vi "AODScanner.vi"() -> ()   [LabVIEW 2011]
uses:
  <vilib>/userdefined/High Color/nirio_resource_hc.ctl
  AODAcq/AODAcq.lvclass
  <vilib>/DAQmx/write.llb/DAQmx Write (Analog DBL 1Chan 1Samp).vi
  <vilib>/DAQmx/read.llb/DAQmx Read (Analog Wfm 1Chan NSamp).vi
  <vilib>/DAQmx/miscellaneous.llb/DAQmx Fill In Error Info.vi
  <vilib>/Utility/error.llb/Error Cluster From Error Code.vi
  <vilib>/rvi/errors/niLvFpgaAdjustHostInterfaceError.vi
  <vilib>/rvi/interface/nirviReadWriteControl/nirviReadWriteControl.xnode
  FPGA_Control/AODRef.ctl
  FPGA_Control/FPGA Bitfiles/AODControl_FPGATarget_5751Acquire_038F9455.lvbitx
  FPGA_Control/AOD Control (FPGA).vi
  NiFpgaLv.dll
panel:
  out "# elements in queue":i32
  out "Waveform Chart":waveform(dbl)(graph)
  out "Ephys":bool
  in  "TraceElements":u32=10000
  out "ScanProgress":dbl(slide) scale=0.0..1.0
  in  "Abort":bool
  out "Progress":dbl(slide) scale=0.0..1.0
  in  "SweepSettings":bool
  in  "stop":bool
  in  "Power":dbl(slide) min=0.0 max=5.0 step=0.1 scale=0.0..2.5
  out "Point Scanning":bool
  out "Volume Scanning":bool
  in  "Tab Control":enum32{"Setup", "Volume", "Traces", "Motion"}(tab)=enum."Volume"
  in  "Ephys":bool
  in  "Motion rate (Hz)":dbl
  in  "ClearPoints":bool
  in  "Recording Settings":T1
  in  "Scan Settings (um)":T2={"XStart"=-100, "XEnd"=100, "XNum"=250, "YStart"=-100, "YEnd"=100, "YNum"=250, "ZStart"=-50, "ZEnd"=50, "ZNum"=30}
  in  "RIO Device":T3="RIO0"
  in  "Objective":enum16{"20x Olympus"}(ring)
  in  "Scan Time (s)":dbl=300.0
  in  "Volume Reps":i32=1 min=1 max=10000
  in  "Volume":bool
  in  "Scan":bool
  in  "Decimate":bool
  out "Motion points":u32
  in  "MaxThreshold":dbl=1.0
  out "Number selected":u32
  in  "Number of cells":u32=200
  in  "Threshold":dbl=0.1
  in  "Max":dbl(slide)=700000.0 scale=0.0..1310720.0
  out "ImCh2":T4(plugin-control)
  out "ImCh1":T4(plugin-control)
  in  "Section":dbl min=0.0 max=29.0 step=1.0
  in  "Segment":bool
  out "Motion Increment":u32
  in  "DisplayVol":bool=TRUE
  out "Motion Ch1":T4(plugin-control)
  out "Ephys":waveform(dbl)[](graph)
  out "Traces":waveform(dbl)[](graph)
  in  "Down Rate":i32=500
  in  "Spacing":dbl=100.0
  out "Motion Ch2":T4(plugin-control)
  out "Finished":bool
  out "Stopped":bool
  out "AODAcq out":refnum<class "AODAcq.lvclass">
  in  "Debug":bool
  in  "GridPoints":u16=10
  out "Scan Settings":T2
  out "VolData":u8[][](array[numeric])
  in  "VolumeElements":u32=10000
  in  "Points":i32[][](array[numeric])
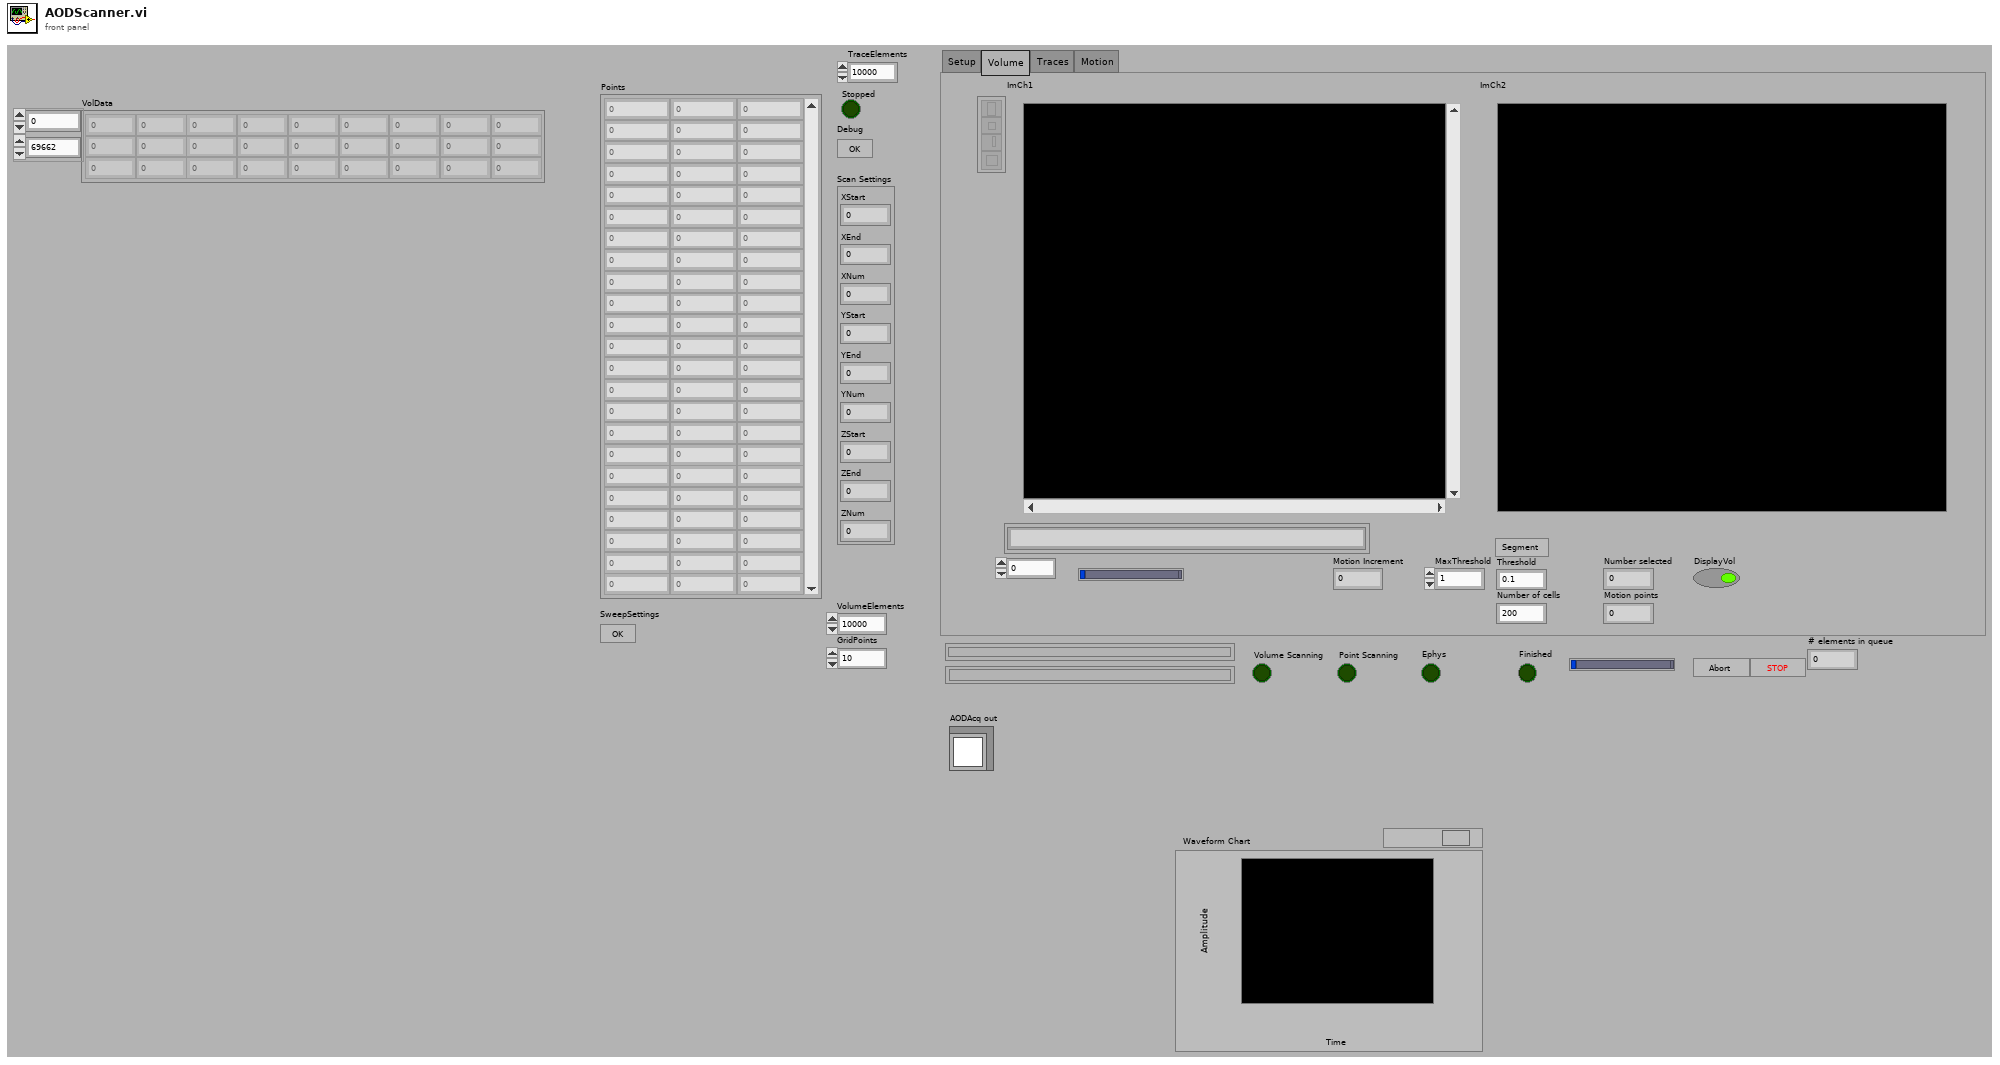
[diagram p1: front panel]
types:
  T1 = cluster{"Path":path, "Save":bool, "SaveRaw":bool}
  T2 = cluster{"XStart":i32, "XEnd":i32, "XNum":i32, "YStart":i32, "YEnd":i32, "YNum":i32, "ZStart":i32, "ZEnd":i32, "ZNum":i32}
  T3 = typedef "nirio_resource_hc.ctl" = tag
  T4 = typedef "IMAQ Image.ctl" = refnum<image>
  T5 = typedef "Image Type" = u32
  T6 = cluster{"Global Rectangle":i32[], "Contours":cluster{"Contour Type":u32, "ROI Type":u32, "Points":i32[]}[]}
  T7 = cluster{"queue out":refnum<queue>, "queue out":refnum<queue>, "queue out":refnum<queue>}
  T8 = typedef "AODRef.ctl" = refnum<k20>
  T9 = cluster{"Global Rectangle":i32[], "Contours":cluster{"Contour Type":u32, "ROI Type":u32, "Points":i32[]}[]}[]
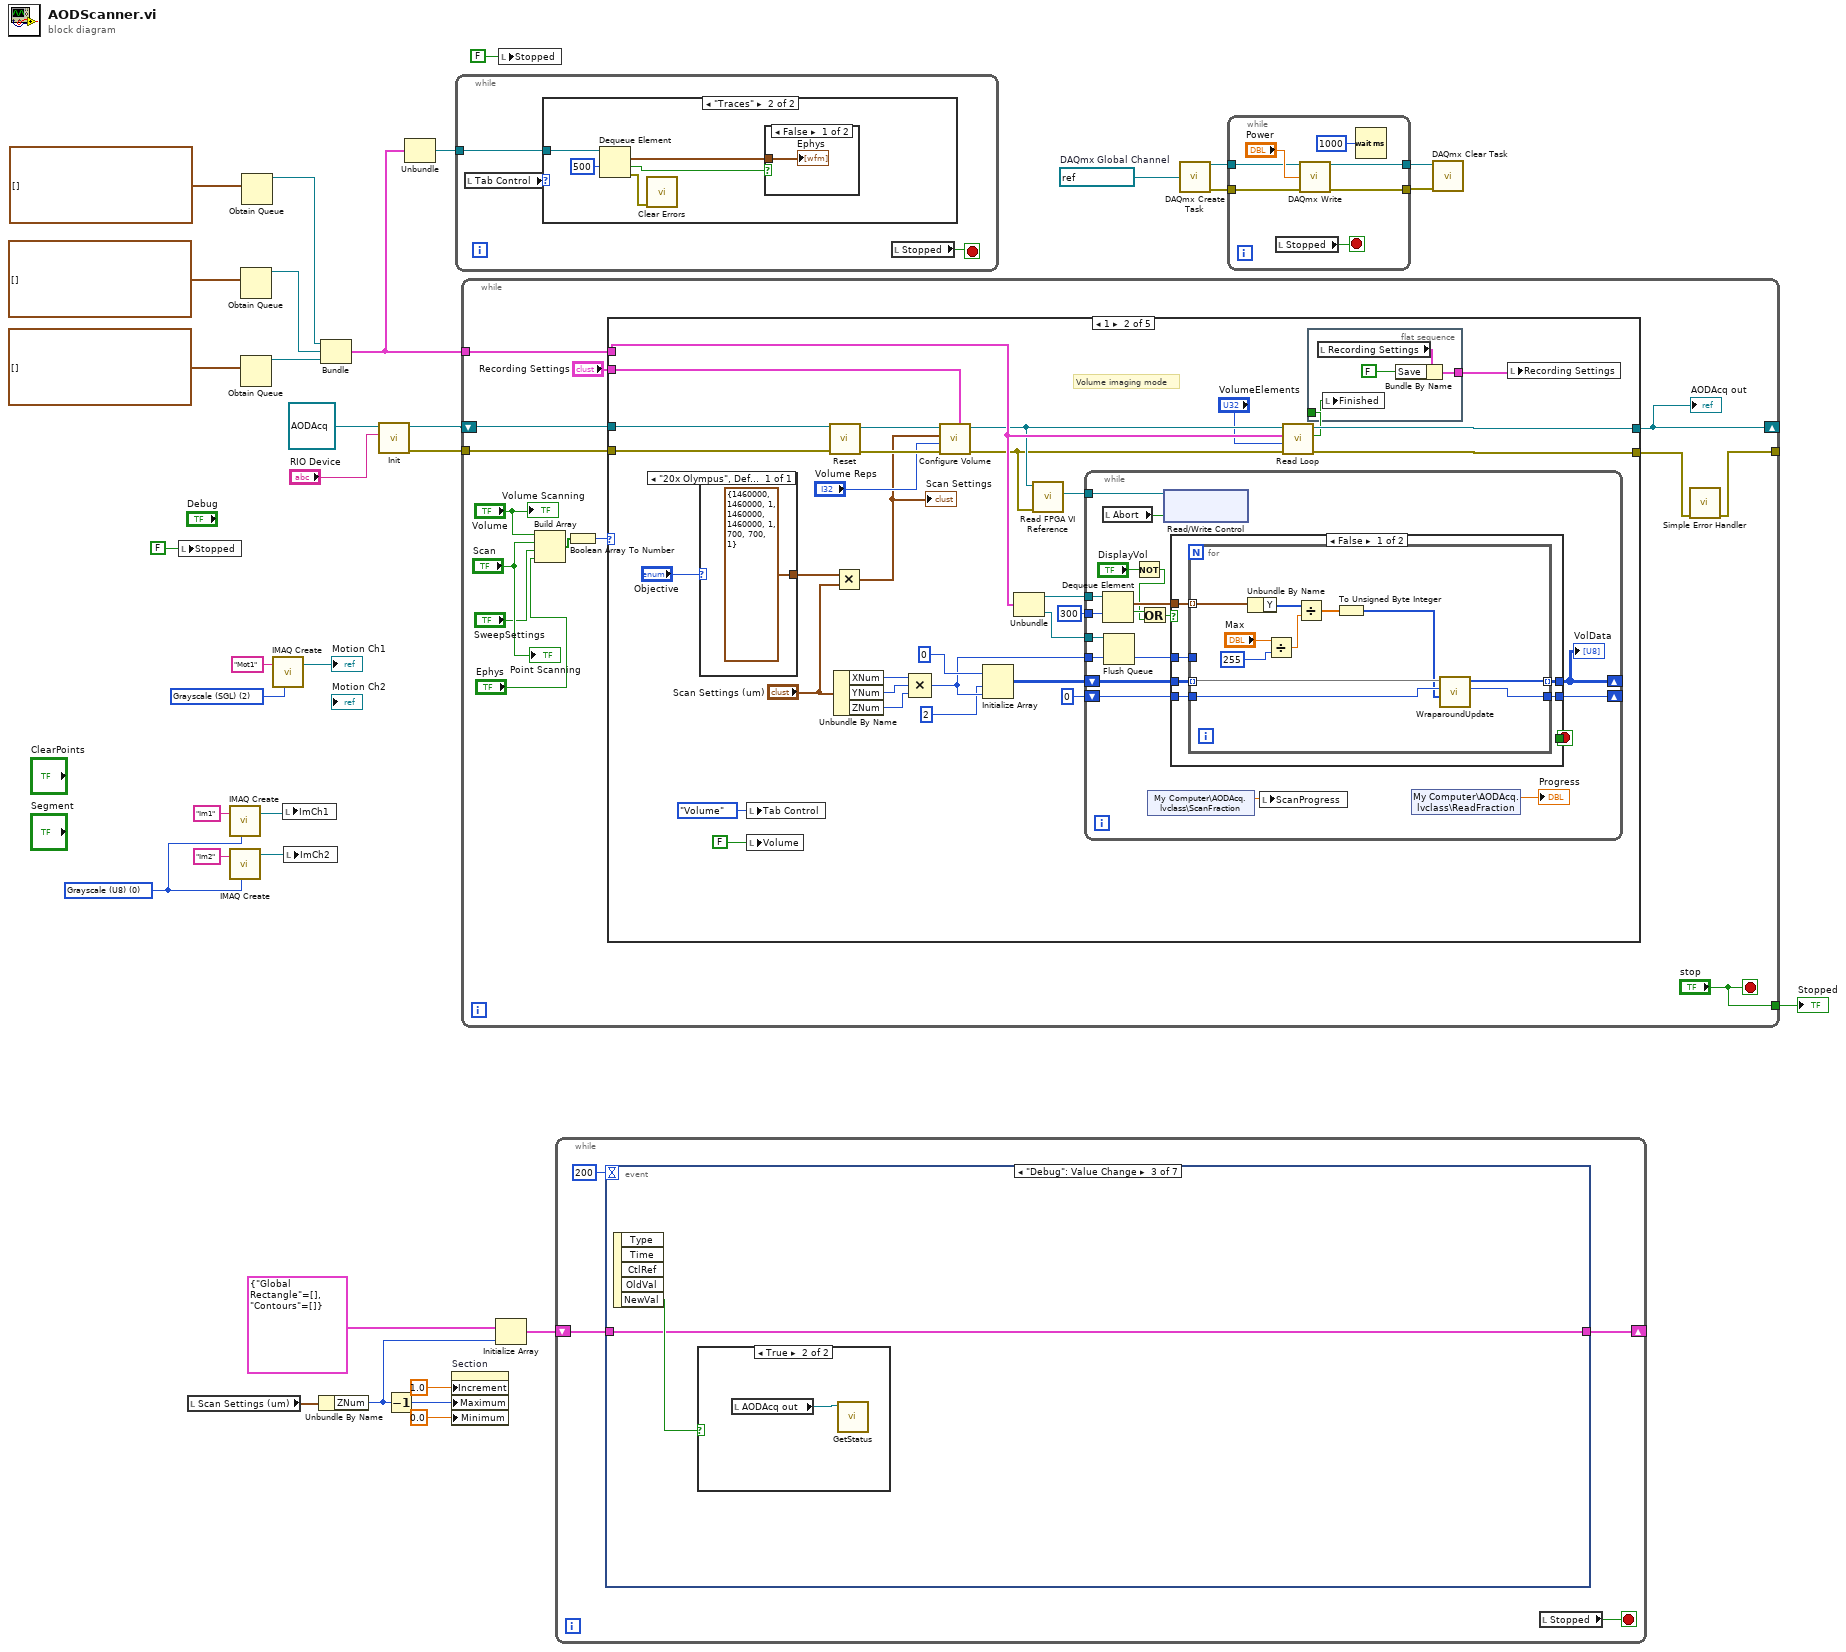
[diagram p0: block diagram]
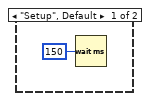
[diagram p2: hidden frame]
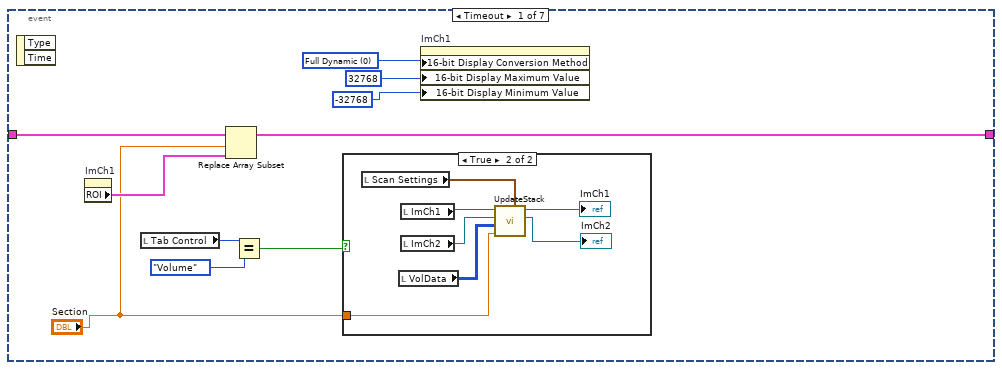
[diagram p4: hidden frame]
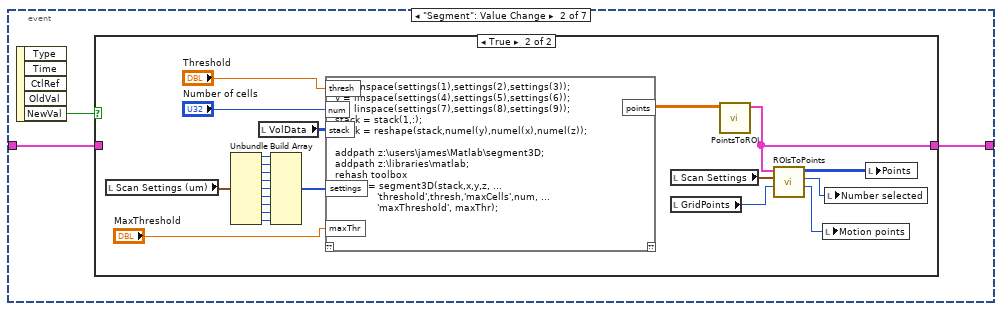
[diagram p6: hidden frame]
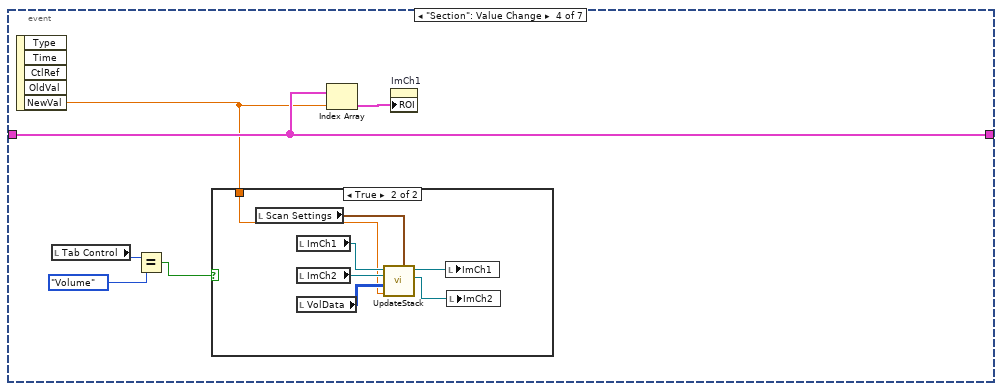
[diagram p9: hidden frame]
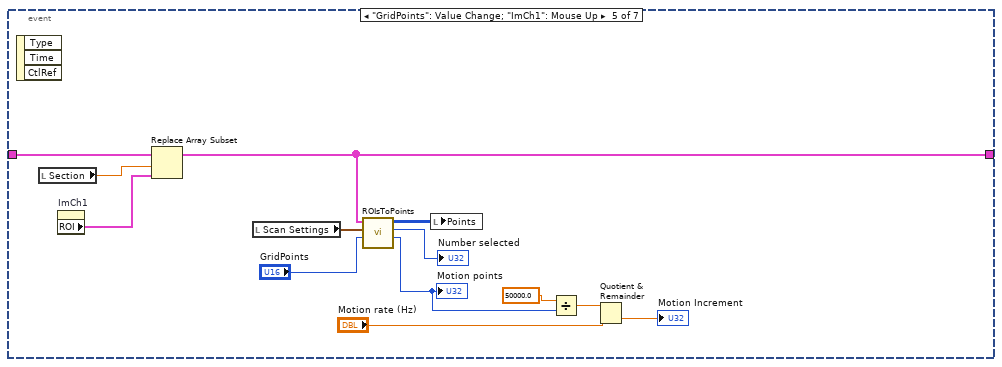
[diagram p11: hidden frame]
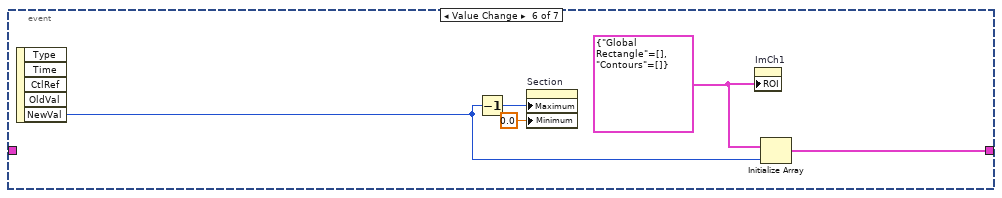
[diagram p12: hidden frame]
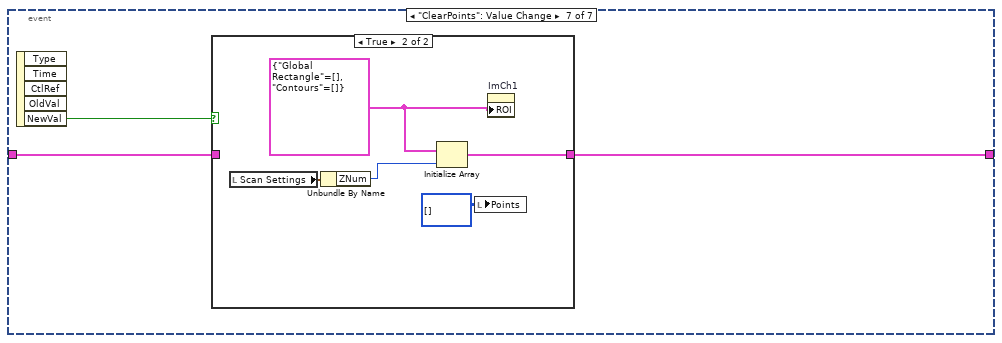
[diagram p13: hidden frame]
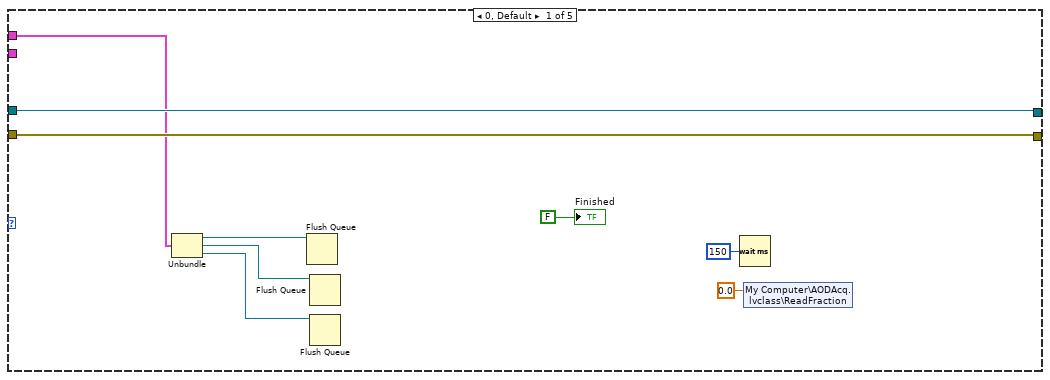
[diagram p15: hidden frame]
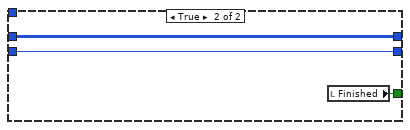
[diagram p16: hidden frame]
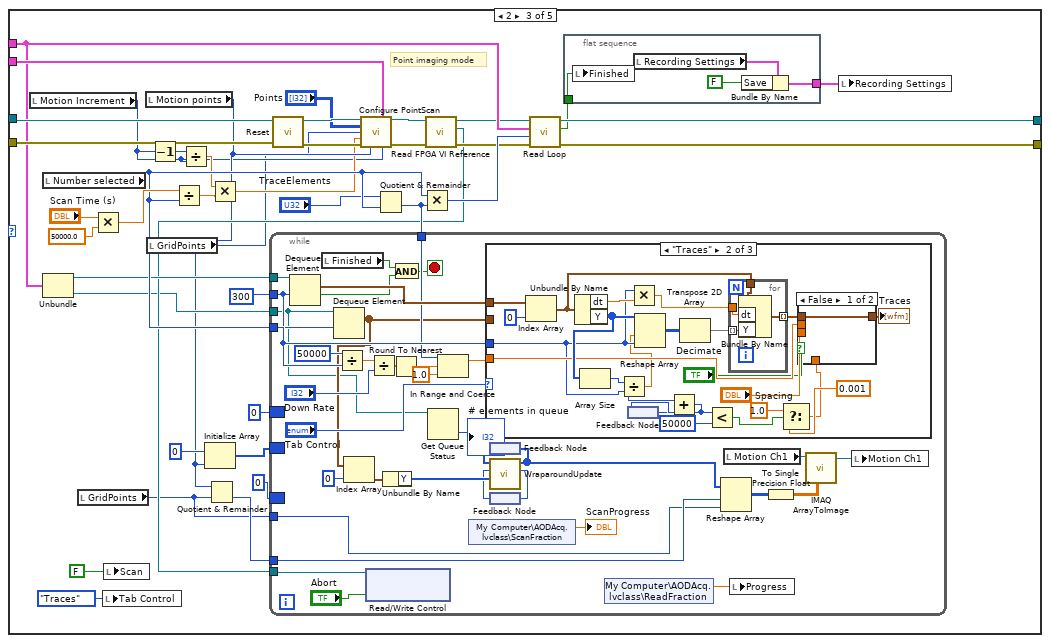
[diagram p17: hidden frame]
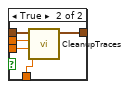
[diagram p19: hidden frame]
diagram:
  w2 = T5 2 items=["Grayscale (U8)", "Grayscale (I16)", "Grayscale (SGL)", "Complex (CSG)", "RGB (U32)", "HSL (U32)", "RGB (U64)", "Grayscale (U16)"] ("Image Type")
  w14 = T5 0 items=["Grayscale (U8)", "Grayscale (I16)", "Grayscale (SGL)", "Complex (CSG)", "RGB (U32)", "HSL (U32)", "RGB (U64)", "Grayscale (U16)"] ("Image Type")
  w26 = refnum<k21> "AOD Gain"  # DAQmx Global Channel
  n1 = local write "Stopped"(FALSE ("Stopped")) -> ()
  n2 = local read "Scan Settings (um)"() -> (w19:T2)
  n3 = call "IMAQ Create"("Image Name"="Im1", "Image Type"=w14) -> ("New Image"=w28:T4)  [unwired: 3 in, 1 out]
  n4 = call "IMAQ Create"("Image Name"="Im2", "Image Type"=w14) -> ("New Image"=w27:T4)  [unwired: 3 in, 1 out]
  n5 = Obtain Queue(element data type=waveform(dbl)[] []) -> (queue out=w9:refnum<queue>)  [unwired: 4 in, 2 out]
  n6 = Obtain Queue(element data type=waveform(i32)[] []) -> (queue out=w7:refnum<queue>)  [unwired: 4 in, 2 out]
  n7 = Obtain Queue(element data type=waveform(i32)[] []) -> (queue out=w8:refnum<queue>)  [unwired: 4 in, 2 out]
  n8 = call "IMAQ Create"("Image Name"="Mot1", "Image Type"=w2) -> ("New Image"=→"Motion Ch1":T4)  [unwired: 3 in, 1 out]
  n9 = local write "ImCh1"(w28) -> ()
  n10 = local write "ImCh2"(w27) -> ()
  n11 = Unbundle By Name(w19) -> ("ZNum"=w13:i32)
  n12 = Bundle("queue out"=w8, "queue out"=w9, "queue out"=w7) -> (w6:T7)  [unwired: 1 in]
  n13 = call "Init.vi"("RIO Device"="RIO Device", "AODAcq in"=refnum<class "AODAcq.lvclass"> refnum ("AODAcq.lvclass")) -> ("error out"=w32:errorcluster, "AODAcq out"=w33:refnum<class "AODAcq.lvclass">)  [unwired: 8 in]
  n14 = Decrement(x=w13) -> (x-1=w12:i32)
  n15 = Unbundle(w6) -> ("queue out"=w5:refnum<queue>)  [unwired: 2 out]
  n16 = property on="Section" class="DigNum (strict)"("Increment"=1.0 ("Data Entry Limits:Increment"), "Maximum"=w12, "Minimum"=0.0 ("Data Entry Limits:Minimum")) -> ()  [unwired: 2 in, 2 out]
  n17 = while {
    tunnel: w5 -> [w38]
    stop <- w37 stop-if-true
    n18 = local read "Tab Control"() -> (w36:enum32{"Setup", "Volume", "Traces", "Motion"})
    n19 = case shown="\"Traces\"" w36 {
      tunnel: w38 -> [_ w44]
      frame "Setup", Default {
        n20 = Wait (ms)(milliseconds to wait=u32 150) -> ()  [unwired: 1 out]
      }
      frame "Traces" {
        n21 = Dequeue Element(queue=w44, timeout in ms (-1)=500) -> (element=w41:waveform(dbl)[], timed out?=w40:bool, error out=w42:errorcluster)  [unwired: 1 in, 1 out]
        n22 = call <vilib>:"Clear Errors.vi"("error in (no error)"=w42) -> ()  [unwired: 6 in, 1 out]
        n23 = case shown="False" w40 {
          tunnel: w41 -> [w45 _]
          frame False {
            "Ephys" <- w45
          }
          frame True {
          }
        }
      }
    }
    n24 = local read "Stopped"() -> (w37:bool)
  }
  n25 = while {
    shift-right: [w51] -> _
    shift-left: w33 -> [w59]
    tunnel: w6 -> [w53]
    tunnel: w32 -> [w58]
    tunnel: [w49] -> _
    tunnel: ["stop"] -> w23
    stop <- "stop" stop-if-true
    n26 = Build Array("Volume", "Scan", "SweepSettings", "Ephys") -> (w55:bool[])
    n27 = Boolean Array To Number(Boolean array=w55) -> (number=w54:u32)
    n28 = case shown="1" w54 {
      tunnel: w59 -> [w64 w100 w184 w261 w284]
      tunnel: w58 -> [w67 w99 w183 w260 _]
      tunnel: [w64 w79 w169 w265 w284] -> w51
      tunnel: [w67 w78 w168 w264 w283] -> w50
      tunnel: w53 -> [w63 w77 w167 _ w286]
      tunnel: "Recording Settings" -> [_ w93 w180 _ _]
      frame 0, Default {
        n29 = Unbundle(w63) -> ("queue out"=w62:refnum<queue>, "queue out"=w61:refnum<queue>, "queue out"=w60:refnum<queue>)
        n30 = Flush Queue(queue=w62) -> ()  [unwired: 1 in, 3 out]
        n31 = Flush Queue(queue=w61) -> ()  [unwired: 1 in, 3 out]
        n32 = Flush Queue(queue=w60) -> ()  [unwired: 1 in, 3 out]
        n33 = Wait (ms)(milliseconds to wait=u32 150) -> ()  [unwired: 1 out]
        n34 = shared-variable "My Computer\\AODAcq.lvclass\\ReadFraction"(0.0 ("ReadFraction")) -> ()  [unwired: 1 in, 1 out]
        "Finished" <- FALSE ("Finished")
      }
      frame 1 {
        # "Volume imaging mode"
        n35 = case shown="\"20x Olympus\", Default" "Objective" {
          tunnel: [T2 {"XStart"=1460000, "XEnd"=1460000, "XNum"=1, "YStart"=1460000, "YEnd"=1460000, "YNum"=1, "ZStart"=700, "ZEnd"=700, "ZNum"=1} ("y")] -> w89
          frame "20x Olympus", Default {
          }
        }
        n36 = local write "Tab Control"(enum32{"Setup", "Volume", "Traces"}."Volume" ("Tab Control")) -> ()
        n37 = local write "Volume"(FALSE ("Volume")) -> ()
        n38 = call-dynamic "Reset.vi"("error in (no error)"=w99, "AODAcq in"=w100) -> ("error out"=w97:errorcluster, "AODAcq out"=w98:refnum<class "AODAcq.lvclass">)  [unwired: 8 in]
        n39 = Multiply(x=w89, y="Scan Settings (um)") -> (x*y=w94:T2)
        "Scan Settings" <- w94
        n40 = Unbundle By Name("Scan Settings (um)") -> ("XNum"=w92:i32, "YNum"=w91:i32, "ZNum"=w90:i32)
        n41 = Compound Arithmetic op=MULTIPLY(w92, w91, w90) -> (w82:i32)
        n42 = call-dynamic "Configure Volume.vi"("Recording Settings"=w93, "error in (no error)"=w97, "NumReps"="Volume Reps", "Scan Settings"=w94, "AODAcq in"=w98) -> ("error out"=w73:errorcluster, "AODAcq out"=w74:refnum<class "AODAcq.lvclass">)  [unwired: 5 in]
        n43 = Initialize Array(u8 0, 2 ("dimension size"), w82) -> (w87:u8[][])
        n44 = Unbundle(w77) -> ("queue out"=w76:refnum<queue>, "queue out"=w69:refnum<queue>)  [unwired: 1 out]
        n45 = call-dynamic "Read FPGA VI Reference.vi"("error in (no error)"=w73, "AODAcq in"=w74) -> ("FPGA VI Reference"=w72:T8)  [unwired: 7 in, 2 out]
        n46 = while {
          tunnel: w76 -> [w122]
          shift-right: [w117] -> _
          shift-left: w87 -> [w121]
          shift-right: [w118] -> _
          shift-left: 0 -> [w119]
          tunnel: w82 -> [w116]
          tunnel: 300 ("timeout in ms (-1)") -> [w115]
          tunnel: w72 -> [w112]
          tunnel: w69 -> [w110]
          stop <- w113 stop-if-true
          n47 = local read "Abort"() -> (w107:bool)
          n48 = Dequeue Element(queue=w122, timeout in ms (-1)=w115) -> (element=w120:waveform(i32)[], timed out?=w109:bool)  [unwired: 1 in, 2 out]
          n49 = Flush Queue(queue=w110) -> ()  [unwired: 1 in, 3 out]
          n50 = Not(x="DisplayVol") -> (.not. x?=w105:bool)
          n51 = Or(x=w109, y=w105) -> (x .or. y?=w108:bool)
          n52 = shared-variable "My Computer\\AODAcq.lvclass\\ScanFraction"() -> (w111:dbl)  [unwired: 1 in, 1 out]
          n53 = xnode "Read/Write Control"("FPGA VI Reference In"=w112, "Control.Abort"=w107) -> ()  [unwired: 1 in, 2 out]
          n54 = case shown="False" w108 {
            tunnel: w121 -> [w128 w142]
            tunnel: w120 -> [w127 _]
            tunnel: w119 -> [w126 w141]
            tunnel: [w125 w141] -> w118
            tunnel: [w124 w142] -> w117
            tunnel: w116 -> [w123 _]
            tunnel: [_ w140] -> w113
            frame False {
              n55 = for {
                tunnel: w128 -> [w132] mode=indexing
                tunnel: w127 -> [w139] mode=indexing
                tunnel: [w133] -> w124 mode=indexing
                tunnel: w126 -> [w130]
                tunnel: [w131] -> w125
                tunnel: w123 -> [_]
                n56 = Unbundle By Name(w139) -> ("Y"=w134:i32[])
                n57 = Divide(x="Max", y=255) -> (x/y=w136:dbl)
                n58 = Divide(x=w134, y=w136) -> (x/y=w135:dbl[])
                n59 = To Unsigned Byte Integer(number=w135) -> (unsigned 8bit integer=w129:u8[])
                n60 = call "WraparoundUpdate.vi"("Data"=w129, "Location"=w130, "Accumulator"=w132) -> ("NewLocation"=w131:u32, "Accumulated"=w133:i32[])  [unwired: 7 in]
              }
            }
            frame True {
              n61 = local read "Finished"() -> (w140:bool)
            }
          }
          "VolData" <- w117
          n62 = local write "ScanProgress"(w111) -> ()
          n63 = shared-variable "My Computer\\AODAcq.lvclass\\ReadFraction"() -> (→"Progress":dbl)  [unwired: 1 in, 1 out]
        }
        n64 = call-dynamic "Read Loop.vi"("error in (no error)"=w73, "ReadElements"="VolumeElements", "Queues"=w77, "AODAcq in"=w74) -> ("error out"=w78:errorcluster, "Done"=w75:bool, "AODAcq out"=w79:refnum<class "AODAcq.lvclass">)  [unwired: 5 in]
        n65 = flat-sequence {
          tunnel: w75 -> [w102]
          tunnel: [w101] -> w71
          frame #0 {
            n66 = local read "Recording Settings"() -> (w104:T1)
            n67 = local write "Finished"(w102) -> ()
            n68 = Bundle By Name(cluster=w104, "Save"=FALSE) -> (w101:T1)
          }
        }
        n69 = local write "Recording Settings"(w71) -> ()
      }
      frame 2 {
        # "Point imaging mode"
        n70 = local read "Motion Increment"() -> (w145:u32)
        n71 = local read "Number selected"() -> (w171:u32)
        n72 = Unbundle(w167) -> ("queue out"=w166:refnum<queue>, "queue out"=w159:refnum<queue>)  [unwired: 1 out]
        n73 = local read "GridPoints"() -> (w157:u16)
        n74 = Multiply(x="Scan Time (s)", y=50000.0) -> (x*y=w176:dbl)
        n75 = local write "Tab Control"(enum32{"Setup", "Volume", "Traces"}."Traces" ("Tab Control")) -> ()
        n76 = local write "Scan"(FALSE ("Scan")) -> ()
        n77 = local read "Motion points"() -> (w154:u32)
        n78 = local read "GridPoints"() -> (w144:u16)
        n79 = Decrement(x=w145) -> (x-1=w147:u32)
        n80 = Divide(x=w176, y=w171) -> (x/y=w149:dbl)
        n81 = Divide(x=w147, y=w145) -> (x/y=w146:dbl)
        n82 = Initialize Array(0 ("element"), w154) -> (w155:i32[])
        n83 = Quotient & Remainder(x=w154, y=w157) -> (floor(x/y)=w158:u32)  [unwired: 1 out]
        n84 = Multiply(x=w146, y=w149) -> (x*y=w148:dbl)
        n85 = call-dynamic "Reset.vi"("error in (no error)"=w183, "AODAcq in"=w184) -> ("error out"=w181:errorcluster, "AODAcq out"=w182:refnum<class "AODAcq.lvclass">)  [unwired: 8 in]
        n86 = call-dynamic "Configure PointScan.vi"("AODAcq in"=w182, "Recording Settings"=w180, "Points"="Points", "GridSize"=w144, "Reps"=w148, "error in (no error)"=w181, "Motion Points"=w154, "Motion Increment"=w145) -> ("AODAcq out"=w163:refnum<class "AODAcq.lvclass">, "error out"=w165:errorcluster)  [unwired: 6 in]
        n87 = Quotient & Remainder(x="TraceElements", y=w171) -> (floor(x/y)=w172:u32)  [unwired: 1 out]
        n88 = Multiply(x=w171, y=w172) -> (x*y=w170:u32)
        n89 = call-dynamic "Read FPGA VI Reference.vi"("error in (no error)"=w165, "AODAcq in"=w163) -> ("error out"=w164:errorcluster, "FPGA VI Reference"=w161:T8, "AODAcq out"=w162:refnum<class "AODAcq.lvclass">)  [unwired: 7 in]
        n90 = while {
          tunnel: w171 -> [w220]
          tunnel: 300 ("timeout in ms (-1)") -> [w207]
          tunnel: w172 -> [w215]
          tunnel: w166 -> [w213]
          tunnel: w161 -> [w212]
          tunnel: w159 -> [w190]
          tunnel: w158 -> [w199]
          tunnel: w157 -> [w198]
          border: w155 -> [_]
          border: 0 -> [_]
          border: 0 -> [_]
          stop <- w210 stop-if-true
          n91 = Dequeue Element(queue=w213, timeout in ms (-1)=w207) -> (element=w224:waveform(i32)[], timed out?=w209:bool)  [unwired: 1 in, 2 out]
          n92 = local read "Finished"() -> (w208:bool)
          n93 = Dequeue Element(queue=w190, timeout in ms (-1)=w207) -> (element=w206:waveform(i32)[])  [unwired: 1 in, 3 out]
          n94 = Divide(x=50000, y=w220) -> (x/y=w219:dbl)
          n95 = Index Array(array=w206, index=0) -> (element=w204:waveform(i32))
          n96 = xnode "Read/Write Control"("FPGA VI Reference In"=w212, "Control.Abort"="Abort") -> ()  [unwired: 1 in, 2 out]
          n97 = Divide(x=w219, y="Down Rate") -> (x/y=w222:dbl)
          n98 = Unbundle By Name(w204) -> ("Y"=w196:i32[])
          n99 = Round To Nearest(number=w222) -> (nearest integer value=w217:dbl)
          n100 = And(x=w208, y=w209) -> (x .and. y?=w210:bool)
          n101 = Get Queue Status(queue=w190) -> (# elements in queue=→"# elements in queue":i32)  [unwired: 2 in, 7 out]
          n102 = In Range and Coerce(upper limit=w215, x=w217, lower limit=1.0) -> (coerced(x)=w214:dbl)  [unwired: 1 out]
          n103 = shared-variable "My Computer\\AODAcq.lvclass\\ScanFraction"() -> (→"ScanProgress":dbl)  [unwired: 1 in, 1 out]
          n104 = case shown="\"Traces\"" "Tab Control" {
            tunnel: w220 -> [_ w237 _]
            tunnel: w224 -> [_ w243 _]
            tunnel: w214 -> [_ w240 _]
            tunnel: w206 -> [_ _ _]
            frame "Setup", Default {
            }
            frame "Traces" {
              n105 = Index Array(array=w243, index=0) -> (element=w244:waveform(i32))
              n106 = Unbundle By Name(w244) -> ("dt"=w246:dbl, "Y"=w242:i32[])
              n107 = Array Size(array=w242) -> (size(s)=w232:i32)
              n108 = Divide(x=w232, y=w237) -> (x/y=w236:dbl)
              n109 = feedback #1() -> (w231:i32)
              n110 = Multiply(x=w237, y=w246) -> (x*y=w245:dbl)
              n111 = Reshape Array(w242, w236, w237) -> (w235:i32[][])
              n112 = Add(x=w232, y=w231) -> (x+y=w227:i32)
              n113 = feedback-in #1(w227) -> ()
              n114 = Transpose 2D Array(2D array=w235) -> (transposed array=w234:i32[][])
              n115 = Less?(x=w227, y=50000) -> (x < y?=w225:bool)
              n116 = for {
                tunnel: w245 -> [w257]
                tunnel: w244 -> [w256]
                tunnel: [w255] -> w239 mode=indexing
                tunnel: w234 -> [w254] mode=indexing
                n117 = Bundle By Name(cluster=w256, "dt"=w257, "Y"=w254) -> (w255:waveform(i32))
              }
              n118 = Select(t=1.0, s=w225, f=0.001 ("Baseline Rate")) -> (s? t:f=w228:dbl)
              n119 = case shown="False" "Decimate" {
                tunnel: "Spacing" -> [_ w253]
                tunnel: w240 -> [_ w252]
                tunnel: w239 -> [w248 w251]
                tunnel: [w248 w250] -> w238
                tunnel: w228 -> [_ w249]
                frame False {
                }
                frame True {
                  n120 = call "CleanupTraces.vi"("Baseline Rate"=w249, "Spacing"=w253, "decimating factor"=w252, "Traces in"=w251) -> ("Traces out"=w250:waveform(dbl)[])  [unwired: 7 in]
                }
              }
              "Traces" <- w238
            }
            frame "Motion" {
            }
          }
          n121 = feedback #2() -> (w195:i32[])
          n122 = feedback #3() -> (w193:u32)
          n123 = call "WraparoundUpdate.vi"("Data"=w196, "Location"=w193, "Accumulator"=w195) -> ("NewLocation"=w194:u32, "Accumulated"=w192:i32[])  [unwired: 7 in]
          n124 = feedback-in #2(w192) -> ()
          n125 = feedback-in #3(w194) -> ()
          n126 = shared-variable "My Computer\\AODAcq.lvclass\\ReadFraction"() -> (w200:dbl)  [unwired: 1 in, 1 out]
          n127 = Reshape Array(w192, w199, w198) -> (w202:i32[][])
          n128 = local read "Motion Ch1"() -> (w201:T4)
          n129 = local write "Progress"(w200) -> ()
          n130 = To Single Precision Float(number=w202) -> (single precision float=w197:sgl[][])
          n131 = call "IMAQ ArrayToImage"("Image Pixels (Float)"=w197, "Image"=w201) -> ("Image Out"=w203:T4)  [unwired: 8 in, 1 out]
          n132 = local write "Motion Ch1"(w203) -> ()
        }
        n133 = call-dynamic "Read Loop.vi"("error in (no error)"=w164, "ReadElements"=w170, "Queues"=w167, "AODAcq in"=w162) -> ("error out"=w168:errorcluster, "Done"=w160:bool, "AODAcq out"=w169:refnum<class "AODAcq.lvclass">)  [unwired: 5 in]
        n134 = flat-sequence {
          tunnel: w160 -> [w186]
          tunnel: [w185] -> w152
          frame #0 {
            n135 = local write "Finished"(w186) -> ()
            n136 = local read "Recording Settings"() -> (w187:T1)
            n137 = Bundle By Name(cluster=w187, "Save"=FALSE) -> (w185:T1)
          }
        }
        n138 = local write "Recording Settings"(w152) -> ()
      }
      frame 4 {
        n139 = call-dynamic "Reset.vi"("error in (no error)"=w260, "AODAcq in"=w261) -> ("error out"=w259:errorcluster, "AODAcq out"=w258:refnum<class "AODAcq.lvclass">)  [unwired: 8 in]
        n140 = call-dynamic "Read FPGA VI Reference.vi"("error in (no error)"=w259, "AODAcq in"=w258) -> ("error out"=w267:errorcluster, "FPGA VI Reference"=w268:T8, "AODAcq out"=w266:refnum<class "AODAcq.lvclass">)  [unwired: 7 in]
        n141 = flat-sequence {
          tunnel: w268 -> [w271]
          tunnel: w267 -> [w269]
          tunnel: w266 -> [w270]
          tunnel: [w270] -> w263
          tunnel: [w269] -> w262
          tunnel: [w273] -> w264
          tunnel: [w272] -> w265
          tunnel: w263 -> [w275]
          tunnel: w262 -> [w274]
          frame #0 {
            n142 = call "SweepSettings.vi"("FPGA VI Reference Out"=w271) -> ()  [unwired: 11 in]
          }
          frame #1 {
            n143 = call-dynamic "GetStatus.vi"("error in (no error)"=w274, "AODAcq in"=w275) -> ("error out"=w273:errorcluster, "AODAcq out"=w272:refnum<class "AODAcq.lvclass">)  [unwired: 7 in, 1 out]
          }
        }
      }
      frame 8 {
        n144 = call "DAQ Assistant"() -> ("task out"=w287:refnum<k21>, "error out"=w282:errorcluster)  [unwired: 16 in, 2 out]
        n145 = local write "Tab Control"(enum32{"Setup", "Volume", "Traces", "Motion"}."Traces" ("Tab Control")) -> ()
        n146 = local write "Ephys"(FALSE ("Ephys")) -> ()
        n147 = Unbundle(w286) -> ("queue out"=w280:refnum<queue>)  [unwired: 2 out]
        n148 = while {
          tunnel: w287 -> [w296]
          tunnel: w280 -> [w295]
          tunnel: [w294] -> w285
          tunnel: w282 -> [w293]
          tunnel: [w291] -> w281
          tunnel: [FALSE ("Ephys")] -> w277
          stop <- w297 stop-if-true
          n149 = call-poly <vilib>:"DAQmx Read.vi"("task/channels in"=w296, "error in"=w293) -> ("task out"=w294:refnum<k21>, "data"=w289:waveform(dbl), "error out"=w292:errorcluster)  [unwired: 11 in]
          "Waveform Chart" <- w289
          n150 = Build Array(w289) -> (w288:waveform(dbl)[])
          n151 = local read "Abort"() -> (w297:bool)
          n152 = Enqueue Element(queue=w295, element=w288, error in (no error)=w292) -> (error out=w291:errorcluster)  [unwired: 1 in, 2 out]
        }
        "Ephys" <- w277
        n153 = local write "Ephys"(TRUE ("Ephys")) -> ()
        n154 = call <vilib>:"DAQmx Clear Task.vi"("task in"=w285, "error in"=w281) -> ("error out"=w283:errorcluster)  [unwired: 13 in]
      }
    }
    "AODAcq out" <- w51
    n155 = call <vilib>:"Simple Error Handler.vi"("error in (no error)"=w50) -> ("error out"=w49:errorcluster)  [unwired: 4 in, 4 out]
    "Volume Scanning" <- "Volume"
    "Point Scanning" <- "Scan"
  }
  "Stopped" <- w23
  n156 = Initialize Array(T6 {"Global Rectangle"=[], "Contours"=[]} ("ROI"), w13) -> (w17:T9)
  n157 = local write "Stopped"(FALSE ("Stopped")) -> ()
  n158 = while {
    shift-right: [w300] -> _
    shift-left: w17 -> [w301]
    stop <- w298 stop-if-true
    n159 = event shown="[2] \"Debug\": Value Change" {
      selector: _ -> [_ _ _ _ _ _ _]
      dyn-events: _ -> [_ _ _ _ _ _ _]
      timeout: 200 -> [_ _ _ _ _ _ _]
      tunnel: w301 -> [w310 w320 w345 w352 w373 _ w379]
      tunnel: [w311 w319 w345 w352 w370 w378 w380] -> w300
      event Timeout {
        w305 = u32 0 items=["Full Dynamic", "Downshift", "Given Range", "90% Dynamic", "Given Percent Range"] ("16-bit Display Mapping:Conversion Method")
        n160 = event-data() -> ()  [unwired: 1 in, 2 out]
        n161 = property on="ImCh1" class="ImageControl"() -> ("ROI"=w309:T6)  [unwired: 2 in, 2 out]
        n162 = local read "Tab Control"() -> (w308:enum32{"Setup", "Volume", "Traces", "Motion"})
        n163 = Replace Array Subset(array=w310, new element=w309, index="Section") -> (w311:T9)
        n164 = Equal?(x=w308, y=enum32{"Setup", "Volume", "Traces"}."Volume") -> (x = y?=w306:bool)
        n165 = case shown="True" w306 {
          tunnel: "Section" -> [_ w312]
          frame False {
          }
          frame True {
            n166 = local read "Scan Settings"() -> (w313:T2)
            n167 = local read "VolData"() -> (w314:u8[][])
            n168 = local read "ImCh1"() -> (w318:T4)
            n169 = local read "ImCh2"() -> (w317:T4)
            n170 = call "UpdateStack.vi"("Scan Settings"=w313, "Section"=w312, "ImData"=w314, "Im2 2"=w317, "Im1 In"=w318) -> ("Im2 Out"=→"ImCh2":T4, "Im1 Out"=→"ImCh1":T4)  [unwired: 5 in]
          }
        }
        n171 = property on="ImCh1" class="ImageControl"("16-bit Display Conversion Method"=w305, "16-bit Display Maximum Value"=32768 ("16-bit Display Mapping:Maximum Value"), "16-bit Display Minimum Value"=-32768 ("16-bit Display Mapping:Maximum Value")) -> ()  [unwired: 2 in, 2 out]
      }
      event "Segment": Value Change {
        n172 = event-data() -> ("NewVal"=w321:bool)  [unwired: 1 in, 4 out]
        n173 = case shown="True" w321 {
          tunnel: w320 -> [w322 _]
          tunnel: [w322 w329] -> w319
          frame False {
          }
          frame True {
            n174 = local read "Scan Settings (um)"() -> (w344:T2)
            n175 = Unbundle(w344) -> ("XStart"=w343:i32, "XEnd"=w342:i32, "XNum"=w341:i32, "YStart"=w340:i32, "YEnd"=w339:i32, "YNum"=w338:i32, "ZStart"=w337:i32, "ZEnd"=w336:i32, "ZNum"=w335:i32)
            n176 = local read "VolData"() -> (w330:u8[][])
            n177 = Build Array(w343, w342, w341, w340, w339, w338, w337, w336, w335) -> (w334:i32[])
            n178 = script code="x = linspace(settings(1),settings(2),settings(3));\ny = linspace(settings(4),settings(5),settings(6));\nz = linspace(settings(7),settings(8),settings(9));\nstack = stack(1,:);\nstack = reshape(stack,numel(y),numel(x),numel(z));\n\naddpath z:\\users\\james\\Matlab\\segment3D;\naddpath z:\\libraries\\matlab;\nrehash toolbox\npoints = segment3D(stack,x,y,z, ...\n              'threshold',thresh,'maxCells',num, ...\n              'maxThreshold', maxThr);"("stack"=w330, "settings"=w334, "num"="Number of cells", "thresh"="Threshold", "maxThr"="MaxThreshold") -> ("points"=w331:cdb[][])  [unwired: 1 in, 1 out]
            n179 = local read "Scan Settings"() -> (w326:T2)
            n180 = local read "GridPoints"() -> (w325:u16)
            n181 = call "PointsToROI.vi"("Points"=w331) -> ("ROIs"=w329:T9)  [unwired: 10 in]
            n182 = call "ROIsToPoints.vi"("GridPoints"=w325, "Scan Settings"=w326, "ROI"=w329) -> ("Number of motion points"=w323:i32, "Number of points"=w327:i32, "Points"=w328:i32[][])  [unwired: 6 in]
            n183 = local write "Motion points"(w323) -> ()
            n184 = local write "Number selected"(w327) -> ()
            n185 = local write "Points"(w328) -> ()
          }
        }
      }
      event "Debug": Value Change {
        n186 = event-data() -> ("NewVal"=w346:bool)  [unwired: 1 in, 4 out]
        n187 = case shown="True" w346 {
          frame False {
          }
          frame True {
            n188 = local read "AODAcq out"() -> (w347:refnum<class "AODAcq.lvclass">)
            n189 = call-dynamic "GetStatus.vi"("AODAcq in"=w347) -> ()  [unwired: 8 in, 3 out]
          }
        }
      }
      event "Section": Value Change {
        n190 = event-data() -> ("NewVal"=w351:dbl)  [unwired: 1 in, 4 out]
        n191 = local read "Tab Control"() -> (w350:enum32{"Setup", "Volume", "Traces", "Motion"})
        n192 = Equal?(x=w350, y=enum32{"Setup", "Volume", "Traces"}."Volume") -> (x = y?=w348:bool)
        n193 = case shown="True" w348 {
          tunnel: w351 -> [_ w355]
          frame False {
          }
          frame True {
            n194 = local read "Scan Settings"() -> (w354:T2)
            n195 = local read "ImCh1"() -> (w358:T4)
            n196 = local read "ImCh2"() -> (w359:T4)
            n197 = local read "VolData"() -> (w360:u8[][])
            n198 = call "UpdateStack.vi"("Scan Settings"=w354, "Section"=w355, "ImData"=w360, "Im2 2"=w359, "Im1 In"=w358) -> ("Im2 Out"=w357:T4, "Im1 Out"=w356:T4)  [unwired: 5 in]
            n199 = local write "ImCh1"(w356) -> ()
            n200 = local write "ImCh2"(w357) -> ()
          }
        }
        n201 = Index Array(array=w352, index=w351) -> (element=w353:T6)
        n202 = property on="ImCh1" class="ImageControl"("ROI"=w353) -> ()  [unwired: 2 in, 2 out]
      }
      event "GridPoints": Value Change; "ImCh1": Mouse Up {
        n203 = event-data() -> ()  [unwired: 1 in, 3 out]
        n204 = local read "Section"() -> (w371:dbl)
        n205 = property on="ImCh1" class="ImageControl"() -> ("ROI"=w372:T6)  [unwired: 2 in, 2 out]
        n206 = Replace Array Subset(array=w373, new element=w372, index=w371) -> (w370:T9)
        n207 = local read "Scan Settings"() -> (w369:T2)
        n208 = call "ROIsToPoints.vi"("GridPoints"="GridPoints", "Scan Settings"=w369, "ROI"=w370) -> ("Number of motion points"=w364:i32, "Number of points"=→"Number selected":i32, "Points"=w367:i32[][])  [unwired: 6 in]
        "Motion points" <- w364
        n209 = local write "Points"(w367) -> ()
        n210 = Divide(x=50000.0, y=w364) -> (x/y=w363:dbl)
        n211 = Quotient & Remainder(x=w363, y="Motion rate (Hz)") -> (floor(x/y)=→"Motion Increment":dbl)  [unwired: 1 out]
      }
      event "Scan Settings (um).ZNum": Value Change {
        w377 = T6 {"Global Rectangle"=[], "Contours"=[]} ("ROI")
        n212 = event-data() -> ("NewVal"=w374:i32)  [unwired: 1 in, 4 out]
        n213 = Decrement(x=w374) -> (x-1=w375:i32)
        n214 = property on="Section" class="DigNum (strict)"("Maximum"=w375, "Minimum"=0.0 ("Data Entry Limits:Minimum")) -> ()  [unwired: 2 in, 2 out]
        n215 = property on="ImCh1" class="ImageControl"("ROI"=w377) -> ()  [unwired: 2 in, 2 out]
        n216 = Initialize Array(w377, w374) -> (w378:T9)
      }
      event "ClearPoints": Value Change {
        n217 = event-data() -> ("NewVal"=w381:bool)  [unwired: 1 in, 4 out]
        n218 = case shown="True" w381 {
          tunnel: [w382 w387] -> w380
          tunnel: w379 -> [w382 _]
          frame False {
          }
          frame True {
            w386 = T6 {"Global Rectangle"=[], "Contours"=[]} ("ROI")
            n219 = local read "Scan Settings"() -> (w385:T2)
            n220 = Unbundle By Name(w385) -> ("ZNum"=w384:i32)
            n221 = Initialize Array(w386, w384) -> (w387:T9)
            n222 = local write "Points"(i32[][] [] ("Points")) -> ()
            n223 = property on="ImCh1" class="ImageControl"("ROI"=w386) -> ()  [unwired: 2 in, 2 out]
          }
        }
      }
    }
    n224 = local read "Stopped"() -> (w298:bool)
  }
  n225 = call <vilib>:"DAQmx Create Task.vi"("global virtual channels"=w26) -> ("task out"=w25:refnum<k21>, "error out"=w24:errorcluster)  [unwired: 4 in, 9 out]
  n226 = while {
    tunnel: w25 -> [w393]
    tunnel: w24 -> [w392]
    tunnel: [w391] -> w22
    tunnel: [w390] -> w21
    stop <- w389 stop-if-true
    n227 = local read "Stopped"() -> (w389:bool)
    n228 = call-poly <vilib>:"DAQmx Write.vi"("task/channels in"=w393, "data"="Power", "error in"=w392) -> ("task out"=w391:refnum<k21>, "error out"=w390:errorcluster)  [unwired: 10 in, 1 out]
    n229 = Wait (ms)(milliseconds to wait=u32 1000) -> ()  [unwired: 1 out]
  }
  n230 = call <vilib>:"DAQmx Clear Task.vi"("task in"=w22, "error in"=w21) -> ()  [unwired: 13 in, 1 out]
